vi "Stop Core.vi"(10 "final error code":i32, 11 "input_poller in":refnum<class "input_poller.lvclass">) -> (3 "input_poller out":refnum<class "input_poller.lvclass">)   [LabVIEW 2015, in "input_poller.lvclass"]
doc: "(<B>Filename</B>: Actor Framework.lvlib:Actor.lvclass:Stop Core.vi)\n\nDefines what the actor does before it stops. Use the <B>final error code</B> input to determine whether the actor shut down in response to an error.\n\nBy default, this method does nothing. A descendant class may override it to define behavior, such as shutting down any processes the actor initiated in its override of the Actor Core method."
uses:
  input_poller.lvclass
  input_poller.lvclass/input_poller.ctl
  <vilib>/ActorFramework/Actor/Actor.lvclass
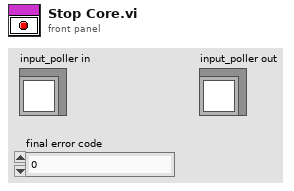
[diagram p1: front panel]
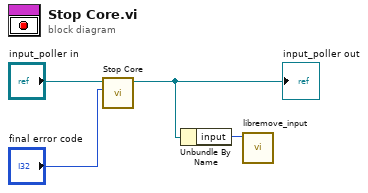
[diagram p0: block diagram]
diagram:
  n1 = call-parent "Stop Core.vi"("final error code"="final error code", "Actor in"="input_poller in") -> ("Actor out"=w1:refnum<class "input_poller.lvclass">)  [unwired: 9 in]
  "input_poller out" <- w1
  n2 = Unbundle By Name(w1) -> ("input"=w2:i32)
  n3 = call "libremove_input.vi"("input"=w2) -> ()  [unwired: 10 in, 1 out]
